vi "Taiko_SGLToPrefix.vi"(11 "SGL":sgl format="%#_12g") -> (2 "PREFIX":string, 3 "MANT":sgl)   [LabVIEW 2017]
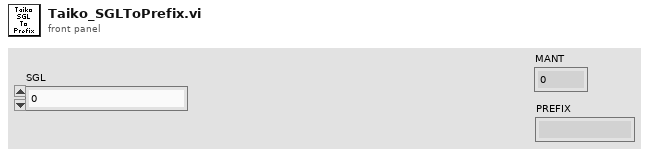
[diagram p1: front panel]
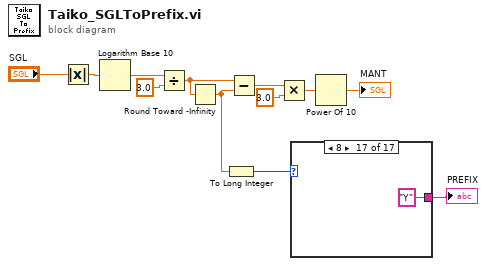
[diagram p0: block diagram]
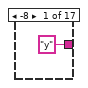
[diagram p2: hidden frame]
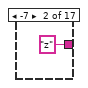
[diagram p3: hidden frame]
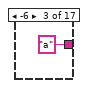
[diagram p4: hidden frame]
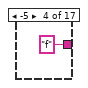
[diagram p5: hidden frame]
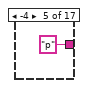
[diagram p6: hidden frame]
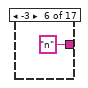
[diagram p7: hidden frame]
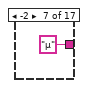
[diagram p8: hidden frame]
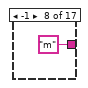
[diagram p9: hidden frame]
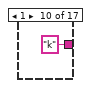
[diagram p11: hidden frame]
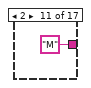
[diagram p12: hidden frame]
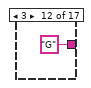
[diagram p13: hidden frame]
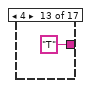
[diagram p14: hidden frame]
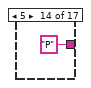
[diagram p15: hidden frame]
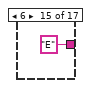
[diagram p16: hidden frame]
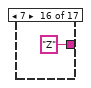
[diagram p17: hidden frame]
diagram:
  n1 = Absolute Value(x="SGL") -> (abs(x)=w11:sgl)
  n2 = Logarithm Base 10(1:w11) -> (0:w9:sgl)
  n3 = Divide(x=w9, y=sgl 3.0) -> (x/y=w6:sgl)
  n4 = Round Toward -Infinity(1:w6) -> (0:w5:sgl)
  n5 = To Long Integer(number=w5) -> (32bit integer=w2:i32)
  n6 = Subtract(x=w6, y=w5) -> (x-y=w4:sgl)
  n7 = Multiply(x=w4, y=sgl 3.0) -> (x*y=w7:sgl)
  n8 = case shown="8" w2 {
    tunnel: ["y" "z" "a" "f" "p" "n" "µ" "m" _ "k" "M" "G" "T" "P" "E" "Z" "Y"] -> w1
    frame -8 {
    }
    frame -7 {
    }
    frame -6 {
    }
    frame -5 {
    }
    frame -4 {
    }
    frame -3 {
    }
    frame -2 {
    }
    frame -1 {
    }
    frame 0, Default {
    }
    frame 1 {
    }
    frame 2 {
    }
    frame 3 {
    }
    frame 4 {
    }
    frame 5 {
    }
    frame 6 {
    }
    frame 7 {
    }
    frame 8 {
    }
  }
  "PREFIX" <- w1
  n9 = Power Of 10(x=w7) -> (10^x=→"MANT":sgl)
